vi "Configure Measurement.vi"(8 "error in (no error)":errorcluster, 10 "Meas Setting":T1={"Function (0: DC Voltage)"=0, "Manual Resolution (5.5 Digits)"=5.5, "Manual Range (1.00)"=1.0, "Enable Auto Range (T: Enable)"=TRUE} {"Manual Range (1.00)" format="%_3f"; "Manual Resolution (5.5 Digits)" items=["4.5"=4.5, "5.5"=5.5, "6.5"=6.5]; "Function (0: DC Voltage)" items=["DC Voltage", "AC Voltage", "2 - Wire Resistance", "4 - Wire Resistance", "DC Current", "AC Current", "Frequency", "Period", "Continuity", "Diode Checking", "VDC:VDC Ratio", "Temperature", "Capacitance"]}, 11 "Abstract in":refnum<class "Abstract.lvclass">) -> (0 "error out":errorcluster, 3 "Abstract out":refnum<class "Abstract.lvclass">)   [LabVIEW 2021, in "DMM.lvlib" / "Abstract.lvclass"]
uses:
  Abstract.lvclass
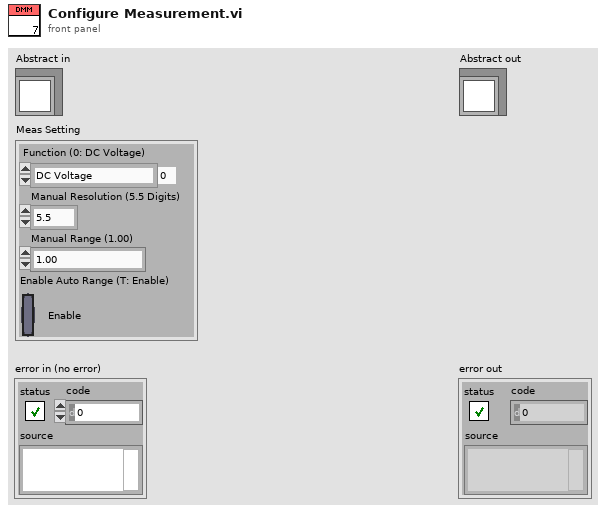
[diagram p1: front panel]
types:
  T1 = cluster{"Function (0: DC Voltage)":u16, "Manual Resolution (5.5 Digits)":dbl, "Manual Range (1.00)":dbl, "Enable Auto Range (T: Enable)":bool}
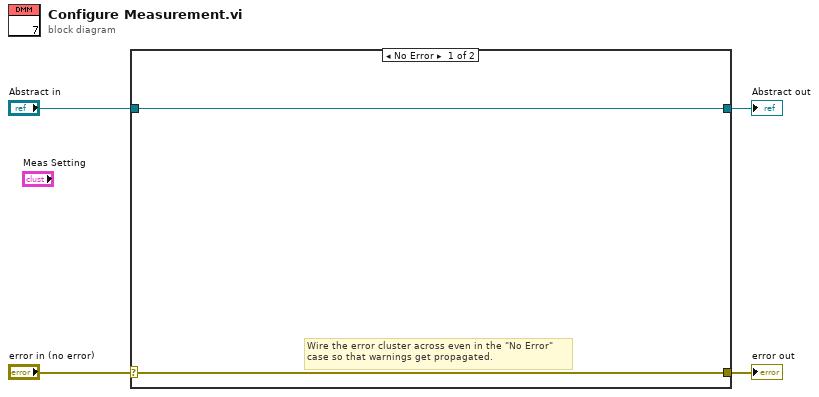
[diagram p0: block diagram]
diagram:
  n1 = case shown="No Error" "error in (no error)" {
    selector: "error in (no error)" -> [w5 w8]
    tunnel: [w5 w8] -> w3
    tunnel: [w6 w7] -> w1
    tunnel: "Abstract in" -> [w6 w7]
    frame No Error {
      # "Wire the error cluster across even in the \"No Error\"\ncase so that warnings get propagated."
    }
    frame Error {
    }
  }
  "error out" <- w3
  "Abstract out" <- w1
